vi "CS4_set.vi"(2 "Action":u16(ring) items=["Up", "Down", "Pause", "Zero"], 3 "Rate in Range (T/min)":dbl[](array[numeric]), 4 "Set Point":dbl, 5 "GPIB add":string) -> (0 "Target B":string, 1 "Rate":string)   [LabVIEW 2012]
panel:
  out "error out":errorcluster
  in  "error in":errorcluster
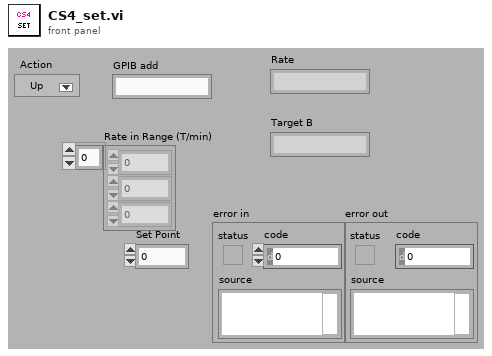
[diagram p1: front panel]
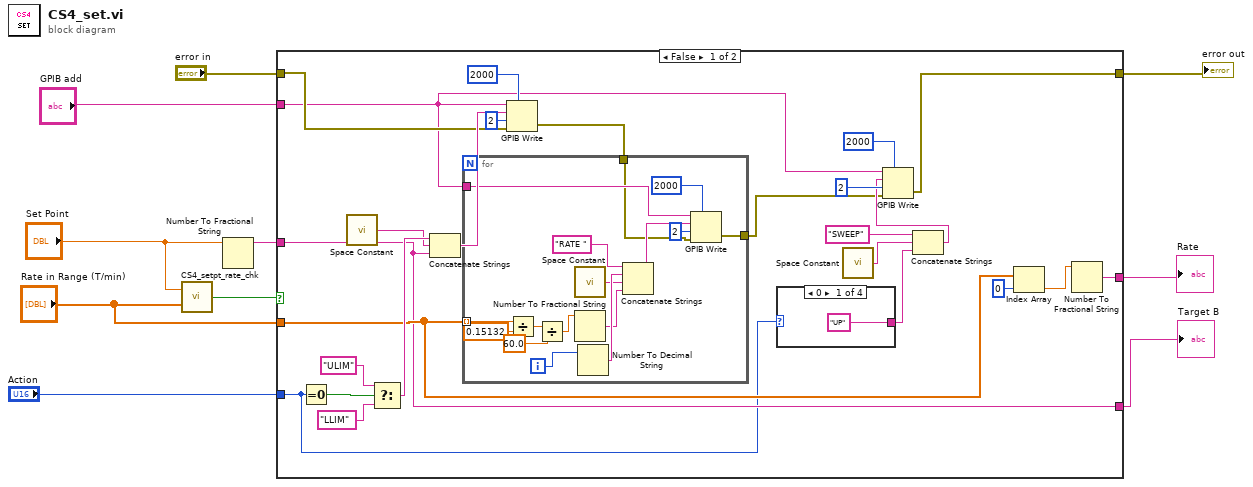
[diagram p0: block diagram]
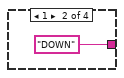
[diagram p2: hidden frame]
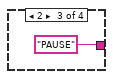
[diagram p3: hidden frame]
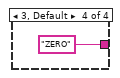
[diagram p4: hidden frame]
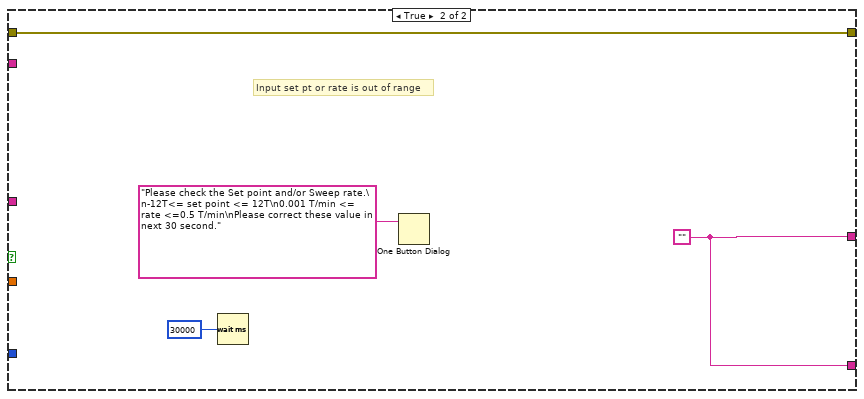
[diagram p5: hidden frame]
diagram:
  n1 = call "CS4_setpt_rate_chk.vi"("Rate in Range (T/min)"="Rate in Range (T/min)", "Set Point"="Set Point") -> ("chk set pt and rate"=w8:bool)
  n2 = Number To Fractional String(number="Set Point") -> (F-format string=w6:string)  [unwired: 3 in]
  n3 = case shown="False" w8 {
    tunnel: "Action" -> [w17 _]
    tunnel: w6 -> [w23 _]
    tunnel: "GPIB add" -> [w18 _]
    tunnel: "Rate in Range (T/min)" -> [w27 _]
    tunnel: "error in" -> [w28 w57]
    tunnel: [w11 w57] -> w4
    tunnel: [w24 w56] -> w2
    tunnel: [w23 w56] -> w1
    frame False {
      n4 = Equal To 0?(x=w17) -> (x = 0?=w35:bool)
      n5 = call <vilib>:"Space Constant.vi"() -> ("String"=w22:string)
      n6 = Select(t="ULIM" ("string"), s=w35, f="LLIM" ("string")) -> (s? t:f=w32:string)
      n7 = Concatenate Strings(w32, w22, w23) -> (w31:string)
      n8 = GPIB Write(0:w18, 1:w31, 2:i16 2 ("mode (0)"), 3:w28, 4:2000 ("timeout ms (488.2 global)")) -> (6:w21:errorcluster)  [unwired: 1 out]
      n9 = for {
        tunnel: w18 -> [w55]
        tunnel: w27 -> [w46] mode=indexing
        tunnel: w21 -> [w41]
        tunnel: [w40] -> w12
        i -> [w52]
        n10 = Divide(x=w46, y=0.15132) -> (x/y=w44:dbl)
        n11 = Divide(x=w44, y=60.0) -> (x/y=w42:dbl)
        n12 = call <vilib>:"Space Constant.vi"() -> ("String"=w50:string)
        n13 = Number To Fractional String(number=w42) -> (F-format string=w49:string)  [unwired: 3 in]
        n14 = Number To Decimal String(number=w52) -> (decimal integer string=w51:string)  [unwired: 1 in]
        n15 = Concatenate Strings("RATE " ("string"), w51, w50, w49) -> (w53:string)
        n16 = GPIB Write(0:w55, 1:w53, 2:i16 2 ("mode (0)"), 3:w41, 4:2000 ("timeout ms (488.2 global)")) -> (6:w40:errorcluster)  [unwired: 1 out]
      }
      n17 = case shown="0" w17 {
        tunnel: ["UP" ("string") "DOWN" ("string") "PAUSE" ("string") "ZERO" ("string")] -> w14
        frame 0 {
        }
        frame 1 {
        }
        frame 2 {
        }
        frame 3, Default {
        }
      }
      n18 = call <vilib>:"Space Constant.vi"() -> ("String"=w15:string)
      n19 = Concatenate Strings("SWEEP" ("string"), w15, w14) -> (w13:string)
      n20 = GPIB Write(0:w18, 1:w13, 2:i16 2 ("mode (0)"), 3:w12, 4:2000 ("timeout ms (488.2 global)")) -> (6:w11:errorcluster)  [unwired: 1 out]
      n21 = Index Array(array=w27, index=0) -> (element=w25:dbl)
      n22 = Number To Fractional String(number=w25) -> (F-format string=w24:string)  [unwired: 3 in]
    }
    frame True {
      w56 = ""
      # "Input set pt or rate is out of range"
      n23 = Wait (ms)(milliseconds to wait=u32 30000) -> ()  [unwired: 1 out]
      n24 = One Button Dialog(message="Please check the Set point and/or Sweep rate.\n-12T<= set point <= 12T\n0.001 T/min <= rate <=0.5 T/min\nPlease correct these value in next 30 second.") -> ()  [unwired: 1 in, 1 out]
    }
  }
  "Rate" <- w2
  "Target B" <- w1
  "error out" <- w4
